vi "10_NET_CALENDARIO_COVID_19_modificado_para_subpanel.vi"() -> ()   [LabVIEW 2019]
uses:
  System.Windows.Forms
panel:
  in  "stop":bool
  in  "OK Button":bool
  out "substring before match":string
  out "date/time string":string
  in  "MonthCalendar 2":refnum<k24>(container)
  in  "MonthCalendar":refnum<k24>(container)
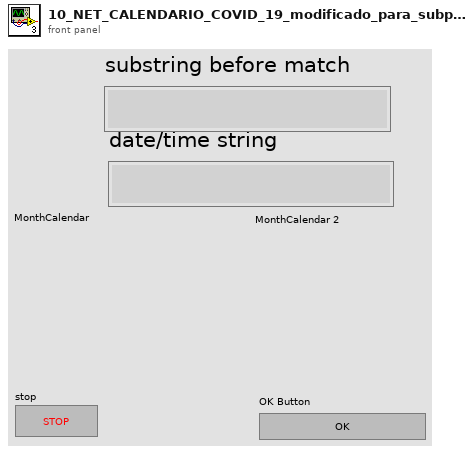
[diagram p1: front panel]
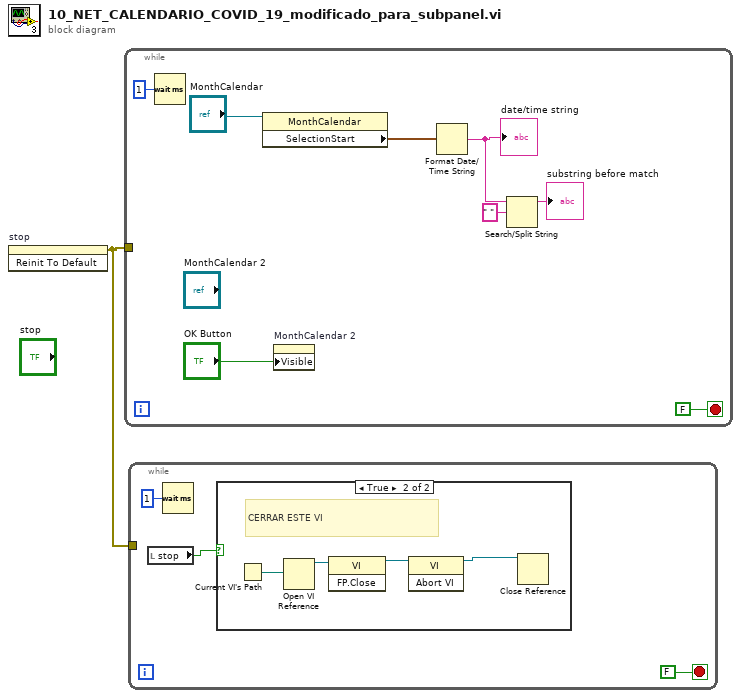
[diagram p0: block diagram]
diagram:
  n1 = invoke on="stop" class="Bool (strict)" method="Reinit To Default"() -> (error out=w1:errorcluster)  [unwired: 3 in, 2 out]
  n2 = while {
    tunnel: w1 -> [_]
    stop <- FALSE stop-if-true
    n3 = Wait (ms)(milliseconds to wait=u32 1) -> ()  [unwired: 1 out]
    n4 = property class="MonthCalendar"(reference="MonthCalendar") -> ("SelectionStart"=w8:timestamp)  [unwired: 1 in, 2 out]
    n5 = property on="MonthCalendar 2" class="AXCont"("Visible"="OK Button") -> ()  [unwired: 2 in, 2 out]
    n6 = Format Date/Time String(seconds (now)=w8) -> (date/time string=w7:string)  [unwired: 2 in]
    "date/time string" <- w7
    n7 = Search/Split String(string=w7, search string/char (-)=" ") -> (substring before match=→"substring before match":string)  [unwired: 1 in, 2 out]
  }
  n8 = while {
    tunnel: w1 -> [_]
    stop <- FALSE stop-if-true
    n9 = local read "stop"() -> (w12:bool)
    n10 = Wait (ms)(milliseconds to wait=u32 1) -> ()  [unwired: 1 out]
    n11 = case shown="True" w12 {
      frame False {
      }
      frame True {
        # "CERRAR ESTE VI"
        n12 = Current VI's Path() -> (path=w16:path)
        n13 = Open VI Reference(vi path=w16) -> (vi reference=w15:refnum<vi>)  [unwired: 5 in, 1 out]
        n14 = invoke class="VI" method="FP.Close"(reference=w15) -> (reference out=w14:refnum<vi>)  [unwired: 2 in, 2 out]
        n15 = invoke class="VI" method="Abort VI"(reference=w14) -> (reference out=w13:refnum<vi>)  [unwired: 2 in, 2 out]
        n16 = Close Reference(reference=w13) -> ()  [unwired: 1 in, 1 out]
      }
    }
  }
